vi "GetAllGObjs.vi"(1 "Prefix":string, 2 "VI":refnum<vi>) -> (0 "GObjs":cluster{"Name":string, "GObj":refnum<vi>}[](array[cluster]))   [LabVIEW 2014]
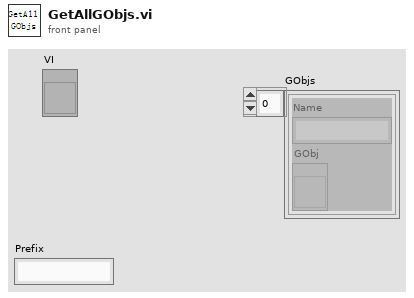
[diagram p1: front panel]
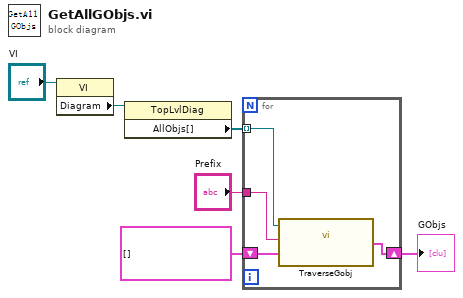
[diagram p0: block diagram]
diagram:
  n1 = property class="VI"(reference="VI") -> ("Diagram"=w6:refnum<vi>)  [unwired: 1 in, 2 out]
  n2 = property class="TopLvlDiag"(reference=w6) -> ("AllObjs[]"=w5:refnum<vi>[])  [unwired: 1 in, 2 out]
  n3 = for {
    tunnel: w5 -> [w10] mode=indexing
    shift-right: [w8] -> w3
    shift-left: cluster{"Name":string, "Ctrl":refnum<vi>}[] [] ("GObjs") -> [w9]
    tunnel: "Prefix" -> [w7]
    n4 = call "TraverseGobj.vi"("Input"=w9, "Prefix"=w7, "GObj Reference"=w10) -> ("Output"=w8:cluster{"Name":string, "Ctrl":refnum<vi>}[])
  }
  "GObjs" <- w3
